vi "Profit Over Time v2.vi"() -> ()   [LabVIEW 2021]
uses:
  35c3a2be-d524-4b83-ae7a-0e43d7c29fc6.vi
  <vilib>/Array/Sort 2D Array - Pop Stack.vi
  <vilib>/Array/Sort 2D Array - Push Stack.vi
  35c3a2be-d524-4b83-ae7a-0e43d7c29fc6.vi/269d4b3b-47f5-49e3-8884-44851e4dd9d5.vi
  35c3a2be-d524-4b83-ae7a-0e43d7c29fc6.vi/6d99389c-673d-4efb-bf33-19b32bcf4cf8.vi
panel:
  in  "Export List?":bool
  in  "Go":bool
  in  "End Date":u16(ring) items=["Mon, Mar 22, 2021", "Mon, Mar 29, 2021", "Mon, Apr 5, 2021", "Mon, Apr 12, 2021", "Mon, Apr 19, 2021", "Mon, Apr 26, 2021", "Mon, May 3, 2021", "Tue, May 4, 2021", "Mon, May 10, 2021", "Mon, May 17, 2021", "Mon, May 24, 2021", "Mon, May 31, 2021", "Mon, Jun 7, 2021", "Mon, Jun 14, 2021", "Mon, Jun 21, 2021", "Mon, Jun 28, 2021", "Mon, Jul 5, 2021", "Mon, Jul 12, 2021", "Mon, Jul 19, 2021", "Mon, Jul 26, 2021", "Mon, Aug 2, 2021", "Mon, Aug 9, 2021", "Mon, Aug 16, 2021", "Mon, Aug 23, 2021", "Mon, Aug 30, 2021", "Mon, Sep 13, 2021", "Mon, Sep 20, 2021", "Mon, Sep 27, 2021", "Mon, Oct 4, 2021", "Mon, Oct 11, 2021", "Mon, Oct 18, 2021", "Mon, Nov 1, 2021", "Mon, Nov 8, 2021", "Mon, Nov 15, 2021", "Wed, Nov 24, 2021", "Mon, Nov 29, 2021", "Mon, Dec 6, 2021", "Mon, Dec 13, 2021", "Tue, Dec 14, 2021", "Wed, Dec 15, 2021", "Thu, Dec 16, 2021", "Fri, Dec 17, 2021", "Sat, Dec 18, 2021", "Mon, Dec 20, 2021", "Tue, Dec 28, 2021", "Wed, Dec 29, 2021", "Thu, Dec 30, 2021", "Fri, Dec 31, 2021", "Sat, Jan 1, 2022", "Sun, Jan 2, 2022", "Mon, Jan 3, 2022", "Tue, Jan 4, 2022", "Wed, Jan 5, 2022", "Thu, Jan 6, 2022", "Fri, Jan 7, 2022", "Sat, Jan 8, 2022", "Sun, Jan 9, 2022", "Mon, Jan 10, 2022", "Thu, Jan 13, 2022", "Sat, Jan 15, 2022", "Sun, Jan 16, 2022", "Mon, Jan 17, 2022", "Fri, Jan 21, 2022", "Mon, Jan 24, 2022", "Wed, Jan 26, 2022", "Thu, Jan 27, 2022", "Fri, Jan 28, 2022", "Sat, Jan 29, 2022", "Mon, Jan 31, 2022", "Wed, Feb 2, 2022", "Thu, Feb 3, 2022", "Mon, Feb 7, 2022", "Tue, Feb 8, 2022", "Wed, Feb 9, 2022", "Thu, Feb 10, 2022", "Fri, Feb 11, 2022", "Mon, Feb 14, 2022", "Tue, Feb 15, 2022", "Wed, Feb 16, 2022", "Thu, Feb 17, 2022", "Sun, Feb 20, 2022", "Mon, Feb 21, 2022", "Tue, Feb 22, 2022", "Wed, Feb 23, 2022", "Thu, Feb 24, 2022", "Fri, Feb 25, 2022", "Sat, Feb 26, 2022", "Sun, Feb 27, 2022", "Mon, Feb 28, 2022", "Fri, Mar 4, 2022", "Sat, Mar 5, 2022", "Sun, Mar 6, 2022", "Mon, Mar 7, 2022", "Tue, Mar 8, 2022", "Wed, Mar 9, 2022", "Fri, Mar 11, 2022", "Sat, Mar 12, 2022", "Sun, Mar 13, 2022", "Mon, Mar 14, 2022", "Wed, Mar 16, 2022", "Sat, Mar 19, 2022", "Sun, Mar 20, 2022", "Mon, Mar 21, 2022", "Tue, Mar 22, 2022", "Wed, Mar 23, 2022", "Thu, Mar 24, 2022", "Fri, Mar 25, 2022", "Sat, Mar 26, 2022", "Sun, Mar 27, 2022", "Mon, Mar 28, 2022", "Tue, Mar 29, 2022", "Wed, Mar 30, 2022", "Thu, Mar 31, 2022", "Sat, Apr 2, 2022", "Mon, Apr 4, 2022", "Sat, Apr 9, 2022", "Sun, Apr 10, 2022", "Mon, Apr 11, 2022", "Tue, Apr 12, 2022", "Wed, Apr 13, 2022", "Sat, Apr 16, 2022", "Sun, Apr 17, 2022", "Mon, Apr 18, 2022", "Thu, Apr 21, 2022", "Sat, Apr 23, 2022", "Sun, Apr 24, 2022", "Mon, Apr 25, 2022", "Tue, Apr 26, 2022", "Thu, Apr 28, 2022", "Fri, Apr 29, 2022", "Sat, Apr 30, 2022", "Mon, May 2, 2022", "Tue, May 3, 2022", "Wed, May 4, 2022", "Thu, May 5, 2022", "Fri, May 6, 2022", "Sat, May 7, 2022", "Sun, May 8, 2022", "Mon, May 9, 2022", "Wed, May 11, 2022", "Thu, May 12, 2022", "Fri, May 13, 2022", "Sat, May 14, 2022", "Sun, May 15, 2022", "Mon, May 16, 2022", "Tue, May 17, 2022", "Thu, May 19, 2022", "Fri, May 20, 2022", "Sat, May 21, 2022", "Sun, May 22, 2022", "Mon, May 23, 2022", "Tue, May 24, 2022", "Wed, May 25, 2022", "Thu, May 26, 2022", "Fri, May 27, 2022", "Sat, May 28, 2022", "Sun, May 29, 2022", "Mon, May 30, 2022", "Tue, May 31, 2022", "Wed, Jun 1, 2022", "Thu, Jun 2, 2022", "Fri, Jun 3, 2022", "Sat, Jun 4, 2022", "Sun, Jun 5, 2022", "Mon, Jun 6, 2022", "Tue, Jun 7, 2022", "Wed, Jun 8, 2022", "Thu, Jun 9, 2022", "Fri, Jun 10, 2022", "Sat, Jun 11, 2022", "Sun, Jun 12, 2022", "Mon, Jun 13, 2022", "Tue, Jun 14, 2022", "Wed, Jun 15, 2022", "Thu, Jun 16, 2022", "Fri, Jun 17, 2022", "Sat, Jun 18, 2022", "Sun, Jun 19, 2022", "Mon, Jun 20, 2022", "Tue, Jun 21, 2022", "Wed, Jun 22, 2022", "Thu, Jun 23, 2022", "Fri, Jun 24, 2022", "Sat, Jun 25, 2022", "Sun, Jun 26, 2022", "Mon, Jun 27, 2022", "Tue, Jun 28, 2022", "Fri, Jul 1, 2022", "Sat, Jul 2, 2022", "Sun, Jul 3, 2022", "Mon, Jul 4, 2022", "Tue, Jul 5, 2022", "Wed, Jul 6, 2022", "Thu, Jul 7, 2022", "Fri, Jul 8, 2022", "Sat, Jul 9, 2022", "Sun, Jul 10, 2022", "Mon, Jul 11, 2022", "Tue, Jul 12, 2022", "Wed, Jul 13, 2022", "Thu, Jul 14, 2022", "Fri, Jul 15, 2022", "Sat, Jul 16, 2022", "Fri, Jul 29, 2022", "Sat, Jul 30, 2022", "Mon, Aug 1, 2022", "Tue, Aug 2, 2022", "Wed, Aug 3, 2022", "Thu, Aug 4, 2022", "Fri, Aug 5, 2022", "Sat, Aug 6, 2022", "Sun, Aug 7, 2022", "Mon, Aug 8, 2022", "Tue, Aug 9, 2022", "Wed, Aug 10, 2022", "Thu, Aug 11, 2022", "Fri, Aug 12, 2022", "Sat, Aug 13, 2022", "Sun, Aug 14, 2022", "Mon, Aug 15, 2022", "Tue, Aug 16, 2022", "Wed, Aug 17, 2022", "Thu, Aug 18, 2022", "Fri, Aug 19, 2022", "Sat, Aug 20, 2022", "Sun, Aug 21, 2022", "Mon, Aug 22, 2022", "Tue, Aug 23, 2022", "Wed, Aug 24, 2022", "Thu, Aug 25, 2022", "Fri, Aug 26, 2022", "Sat, Aug 27, 2022", "Sun, Aug 28, 2022", "Mon, Aug 29, 2022", "Tue, Aug 30, 2022", "Wed, Aug 31, 2022", "Thu, Sep 1, 2022", "Fri, Sep 2, 2022", "Sat, Sep 3, 2022", "Sun, Sep 4, 2022", "Mon, Sep 5, 2022", "Tue, Sep 6, 2022", "Wed, Sep 7, 2022", "Sat, Sep 10, 2022", "Sun, Sep 11, 2022", "Mon, Sep 12, 2022", "Tue, Sep 13, 2022", "Wed, Sep 14, 2022", "Thu, Sep 15, 2022", "Fri, Sep 16, 2022", "Sat, Sep 17, 2022", "Sun, Sep 18, 2022", "Mon, Sep 19, 2022", "Tue, Sep 20, 2022", "Wed, Sep 21, 2022", "Thu, Sep 22, 2022", "Fri, Sep 23, 2022", "Sat, Sep 24, 2022", "Sun, Sep 25, 2022", "Mon, Sep 26, 2022", "Tue, Sep 27, 2022", "Wed, Sep 28, 2022", "Thu, Sep 29, 2022", "Fri, Sep 30, 2022", "Sat, Oct 1, 2022", "Mon, Oct 3, 2022", "Wed, Oct 5, 2022", "Thu, Oct 6, 2022", "Fri, Oct 7, 2022", "Sat, Oct 8, 2022", "Mon, Oct 10, 2022", "Wed, Oct 12, 2022", "Thu, Oct 13, 2022", "Fri, Oct 14, 2022", "Sat, Oct 15, 2022", "Mon, Oct 17, 2022", "Tue, Oct 18, 2022", "Wed, Oct 19, 2022", "Thu, Oct 20, 2022", "Fri, Oct 21, 2022", "Sat, Oct 22, 2022", "Sun, Oct 23, 2022", "Mon, Oct 24, 2022", "Tue, Oct 25, 2022", "Wed, Oct 26, 2022", "Thu, Oct 27, 2022", "Fri, Oct 28, 2022", "Sat, Oct 29, 2022", "Mon, Oct 31, 2022", "Tue, Nov 1, 2022", "Wed, Nov 2, 2022", "Thu, Nov 3, 2022", "Fri, Nov 4, 2022", "Sat, Nov 5, 2022", "Sun, Nov 6, 2022", "Mon, Nov 7, 2022", "Wed, Nov 9, 2022", "Thu, Nov 10, 2022", "Fri, Nov 11, 2022", "Sat, Nov 12, 2022", "Sun, Nov 13, 2022", "Mon, Nov 14, 2022", "Tue, Nov 15, 2022", "Thu, Nov 17, 2022", "Fri, Nov 18, 2022", "Sat, Nov 19, 2022", "Mon, Nov 21, 2022", "Tue, Nov 22, 2022", "Wed, Nov 23, 2022", "Thu, Nov 24, 2022", "Fri, Nov 25, 2022", "Sat, Nov 26, 2022", "Sun, Nov 27, 2022", "Mon, Nov 28, 2022", "Tue, Nov 29, 2022", "Wed, Nov 30, 2022", "Thu, Dec 1, 2022", "Fri, Dec 2, 2022", "Tue, Dec 13, 2022", "Wed, Dec 14, 2022", "Thu, Dec 15, 2022", "Fri, Dec 16, 2022", "Sat, Dec 17, 2022", "Sun, Dec 18, 2022", "Mon, Dec 19, 2022", "Tue, Dec 20, 2022", "Wed, Dec 21, 2022", "Thu, Dec 22, 2022", "Fri, Dec 23, 2022", "Sat, Dec 24, 2022", "Sun, Dec 25, 2022", "Mon, Dec 26, 2022", "Tue, Dec 27, 2022", "Wed, Dec 28, 2022", "Thu, Dec 29, 2022", "Fri, Dec 30, 2022", "Sat, Dec 31, 2022", "Sun, Jan 1, 2023", "Mon, Jan 2, 2023"]
  in  "Start Date":u16(ring) items=["Mon, Mar 22, 2021", "Mon, Mar 29, 2021", "Mon, Apr 5, 2021", "Mon, Apr 12, 2021", "Mon, Apr 19, 2021", "Mon, Apr 26, 2021", "Mon, May 3, 2021", "Tue, May 4, 2021", "Mon, May 10, 2021", "Mon, May 17, 2021", "Mon, May 24, 2021", "Mon, May 31, 2021", "Mon, Jun 7, 2021", "Mon, Jun 14, 2021", "Mon, Jun 21, 2021", "Mon, Jun 28, 2021", "Mon, Jul 5, 2021", "Mon, Jul 12, 2021", "Mon, Jul 19, 2021", "Mon, Jul 26, 2021", "Mon, Aug 2, 2021", "Mon, Aug 9, 2021", "Mon, Aug 16, 2021", "Mon, Aug 23, 2021", "Mon, Aug 30, 2021", "Mon, Sep 13, 2021", "Mon, Sep 20, 2021", "Mon, Sep 27, 2021", "Mon, Oct 4, 2021", "Mon, Oct 11, 2021", "Mon, Oct 18, 2021", "Mon, Nov 1, 2021", "Mon, Nov 8, 2021", "Mon, Nov 15, 2021", "Wed, Nov 24, 2021", "Mon, Nov 29, 2021", "Mon, Dec 6, 2021", "Mon, Dec 13, 2021", "Tue, Dec 14, 2021", "Wed, Dec 15, 2021", "Thu, Dec 16, 2021", "Fri, Dec 17, 2021", "Sat, Dec 18, 2021", "Mon, Dec 20, 2021", "Tue, Dec 28, 2021", "Wed, Dec 29, 2021", "Thu, Dec 30, 2021", "Fri, Dec 31, 2021", "Sat, Jan 1, 2022", "Sun, Jan 2, 2022", "Mon, Jan 3, 2022", "Tue, Jan 4, 2022", "Wed, Jan 5, 2022", "Thu, Jan 6, 2022", "Fri, Jan 7, 2022", "Sat, Jan 8, 2022", "Sun, Jan 9, 2022", "Mon, Jan 10, 2022", "Thu, Jan 13, 2022", "Sat, Jan 15, 2022", "Sun, Jan 16, 2022", "Mon, Jan 17, 2022", "Fri, Jan 21, 2022", "Mon, Jan 24, 2022", "Wed, Jan 26, 2022", "Thu, Jan 27, 2022", "Fri, Jan 28, 2022", "Sat, Jan 29, 2022", "Mon, Jan 31, 2022", "Wed, Feb 2, 2022", "Thu, Feb 3, 2022", "Mon, Feb 7, 2022", "Tue, Feb 8, 2022", "Wed, Feb 9, 2022", "Thu, Feb 10, 2022", "Fri, Feb 11, 2022", "Mon, Feb 14, 2022", "Tue, Feb 15, 2022", "Wed, Feb 16, 2022", "Thu, Feb 17, 2022", "Sun, Feb 20, 2022", "Mon, Feb 21, 2022", "Tue, Feb 22, 2022", "Wed, Feb 23, 2022", "Thu, Feb 24, 2022", "Fri, Feb 25, 2022", "Sat, Feb 26, 2022", "Sun, Feb 27, 2022", "Mon, Feb 28, 2022", "Fri, Mar 4, 2022", "Sat, Mar 5, 2022", "Sun, Mar 6, 2022", "Mon, Mar 7, 2022", "Tue, Mar 8, 2022", "Wed, Mar 9, 2022", "Fri, Mar 11, 2022", "Sat, Mar 12, 2022", "Sun, Mar 13, 2022", "Mon, Mar 14, 2022", "Wed, Mar 16, 2022", "Sat, Mar 19, 2022", "Sun, Mar 20, 2022", "Mon, Mar 21, 2022", "Tue, Mar 22, 2022", "Wed, Mar 23, 2022", "Thu, Mar 24, 2022", "Fri, Mar 25, 2022", "Sat, Mar 26, 2022", "Sun, Mar 27, 2022", "Mon, Mar 28, 2022", "Tue, Mar 29, 2022", "Wed, Mar 30, 2022", "Thu, Mar 31, 2022", "Sat, Apr 2, 2022", "Mon, Apr 4, 2022", "Sat, Apr 9, 2022", "Sun, Apr 10, 2022", "Mon, Apr 11, 2022", "Tue, Apr 12, 2022", "Wed, Apr 13, 2022", "Sat, Apr 16, 2022", "Sun, Apr 17, 2022", "Mon, Apr 18, 2022", "Thu, Apr 21, 2022", "Sat, Apr 23, 2022", "Sun, Apr 24, 2022", "Mon, Apr 25, 2022", "Tue, Apr 26, 2022", "Thu, Apr 28, 2022", "Fri, Apr 29, 2022", "Sat, Apr 30, 2022", "Mon, May 2, 2022", "Tue, May 3, 2022", "Wed, May 4, 2022", "Thu, May 5, 2022", "Fri, May 6, 2022", "Sat, May 7, 2022", "Sun, May 8, 2022", "Mon, May 9, 2022", "Wed, May 11, 2022", "Thu, May 12, 2022", "Fri, May 13, 2022", "Sat, May 14, 2022", "Sun, May 15, 2022", "Mon, May 16, 2022", "Tue, May 17, 2022", "Thu, May 19, 2022", "Fri, May 20, 2022", "Sat, May 21, 2022", "Sun, May 22, 2022", "Mon, May 23, 2022", "Tue, May 24, 2022", "Wed, May 25, 2022", "Thu, May 26, 2022", "Fri, May 27, 2022", "Sat, May 28, 2022", "Sun, May 29, 2022", "Mon, May 30, 2022", "Tue, May 31, 2022", "Wed, Jun 1, 2022", "Thu, Jun 2, 2022", "Fri, Jun 3, 2022", "Sat, Jun 4, 2022", "Sun, Jun 5, 2022", "Mon, Jun 6, 2022", "Tue, Jun 7, 2022", "Wed, Jun 8, 2022", "Thu, Jun 9, 2022", "Fri, Jun 10, 2022", "Sat, Jun 11, 2022", "Sun, Jun 12, 2022", "Mon, Jun 13, 2022", "Tue, Jun 14, 2022", "Wed, Jun 15, 2022", "Thu, Jun 16, 2022", "Fri, Jun 17, 2022", "Sat, Jun 18, 2022", "Sun, Jun 19, 2022", "Mon, Jun 20, 2022", "Tue, Jun 21, 2022", "Wed, Jun 22, 2022", "Thu, Jun 23, 2022", "Fri, Jun 24, 2022", "Sat, Jun 25, 2022", "Sun, Jun 26, 2022", "Mon, Jun 27, 2022", "Tue, Jun 28, 2022", "Fri, Jul 1, 2022", "Sat, Jul 2, 2022", "Sun, Jul 3, 2022", "Mon, Jul 4, 2022", "Tue, Jul 5, 2022", "Wed, Jul 6, 2022", "Thu, Jul 7, 2022", "Fri, Jul 8, 2022", "Sat, Jul 9, 2022", "Sun, Jul 10, 2022", "Mon, Jul 11, 2022", "Tue, Jul 12, 2022", "Wed, Jul 13, 2022", "Thu, Jul 14, 2022", "Fri, Jul 15, 2022", "Sat, Jul 16, 2022", "Fri, Jul 29, 2022", "Sat, Jul 30, 2022", "Mon, Aug 1, 2022", "Tue, Aug 2, 2022", "Wed, Aug 3, 2022", "Thu, Aug 4, 2022", "Fri, Aug 5, 2022", "Sat, Aug 6, 2022", "Sun, Aug 7, 2022", "Mon, Aug 8, 2022", "Tue, Aug 9, 2022", "Wed, Aug 10, 2022", "Thu, Aug 11, 2022", "Fri, Aug 12, 2022", "Sat, Aug 13, 2022", "Sun, Aug 14, 2022", "Mon, Aug 15, 2022", "Tue, Aug 16, 2022", "Wed, Aug 17, 2022", "Thu, Aug 18, 2022", "Fri, Aug 19, 2022", "Sat, Aug 20, 2022", "Sun, Aug 21, 2022", "Mon, Aug 22, 2022", "Tue, Aug 23, 2022", "Wed, Aug 24, 2022", "Thu, Aug 25, 2022", "Fri, Aug 26, 2022", "Sat, Aug 27, 2022", "Sun, Aug 28, 2022", "Mon, Aug 29, 2022", "Tue, Aug 30, 2022", "Wed, Aug 31, 2022", "Thu, Sep 1, 2022", "Fri, Sep 2, 2022", "Sat, Sep 3, 2022", "Sun, Sep 4, 2022", "Mon, Sep 5, 2022", "Tue, Sep 6, 2022", "Wed, Sep 7, 2022", "Sat, Sep 10, 2022", "Sun, Sep 11, 2022", "Mon, Sep 12, 2022", "Tue, Sep 13, 2022", "Wed, Sep 14, 2022", "Thu, Sep 15, 2022", "Fri, Sep 16, 2022", "Sat, Sep 17, 2022", "Sun, Sep 18, 2022", "Mon, Sep 19, 2022", "Tue, Sep 20, 2022", "Wed, Sep 21, 2022", "Thu, Sep 22, 2022", "Fri, Sep 23, 2022", "Sat, Sep 24, 2022", "Sun, Sep 25, 2022", "Mon, Sep 26, 2022", "Tue, Sep 27, 2022", "Wed, Sep 28, 2022", "Thu, Sep 29, 2022", "Fri, Sep 30, 2022", "Sat, Oct 1, 2022", "Mon, Oct 3, 2022", "Wed, Oct 5, 2022", "Thu, Oct 6, 2022", "Fri, Oct 7, 2022", "Sat, Oct 8, 2022", "Mon, Oct 10, 2022", "Wed, Oct 12, 2022", "Thu, Oct 13, 2022", "Fri, Oct 14, 2022", "Sat, Oct 15, 2022", "Mon, Oct 17, 2022", "Tue, Oct 18, 2022", "Wed, Oct 19, 2022", "Thu, Oct 20, 2022", "Fri, Oct 21, 2022", "Sat, Oct 22, 2022", "Sun, Oct 23, 2022", "Mon, Oct 24, 2022", "Tue, Oct 25, 2022", "Wed, Oct 26, 2022", "Thu, Oct 27, 2022", "Fri, Oct 28, 2022", "Sat, Oct 29, 2022", "Mon, Oct 31, 2022", "Tue, Nov 1, 2022", "Wed, Nov 2, 2022", "Thu, Nov 3, 2022", "Fri, Nov 4, 2022", "Sat, Nov 5, 2022", "Sun, Nov 6, 2022", "Mon, Nov 7, 2022", "Wed, Nov 9, 2022", "Thu, Nov 10, 2022", "Fri, Nov 11, 2022", "Sat, Nov 12, 2022", "Sun, Nov 13, 2022", "Mon, Nov 14, 2022", "Tue, Nov 15, 2022", "Thu, Nov 17, 2022", "Fri, Nov 18, 2022", "Sat, Nov 19, 2022", "Mon, Nov 21, 2022", "Tue, Nov 22, 2022", "Wed, Nov 23, 2022", "Thu, Nov 24, 2022", "Fri, Nov 25, 2022", "Sat, Nov 26, 2022", "Sun, Nov 27, 2022", "Mon, Nov 28, 2022", "Tue, Nov 29, 2022", "Wed, Nov 30, 2022", "Thu, Dec 1, 2022", "Fri, Dec 2, 2022", "Tue, Dec 13, 2022", "Wed, Dec 14, 2022", "Thu, Dec 15, 2022", "Fri, Dec 16, 2022", "Sat, Dec 17, 2022", "Sun, Dec 18, 2022", "Mon, Dec 19, 2022", "Tue, Dec 20, 2022", "Wed, Dec 21, 2022", "Thu, Dec 22, 2022", "Fri, Dec 23, 2022", "Sat, Dec 24, 2022", "Sun, Dec 25, 2022", "Mon, Dec 26, 2022", "Tue, Dec 27, 2022", "Wed, Dec 28, 2022", "Thu, Dec 29, 2022", "Fri, Dec 30, 2022", "Sat, Dec 31, 2022", "Sun, Jan 1, 2023", "Mon, Jan 2, 2023"]
  out "Complete List":cluster{"Player Name":string, "Profit":dbl}[](array[cluster])
  out "Top 5":cluster{"Player Name":string, "Profit":dbl}[](array[cluster])
  out "residual":dbl
  in  "file path (use dialog)":path=path "C:/Users/manma/Google Drive/WPC Stat Scrape/Data/WPC Stats.bin"
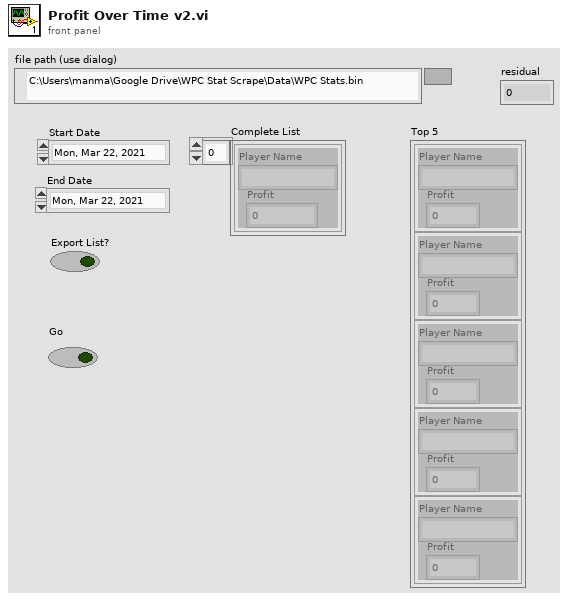
[diagram p1: front panel]
types:
  T1 = typedef "WPC Player and Financial Stats.ctl" = cluster{"Player Name":string, "Date Updated":timestamp, "Tournament Stats":cluster{"Hands Won":i32, "Hands Played":i32, "Hands Dealt":i32, "All-Ins":i32, "Entered":i32, "Winnings":dbl, "Profit":dbl}, "Cash Stats":cluster{"Hands Won":i32, "Hands Played":i32, "Hands Dealt":i32, "All-Ins":i32, "Profit":dbl}}
  T2 = enum16{"open", "replace", "create", "open or create", "replace or create", "replace or create with confirmation"}
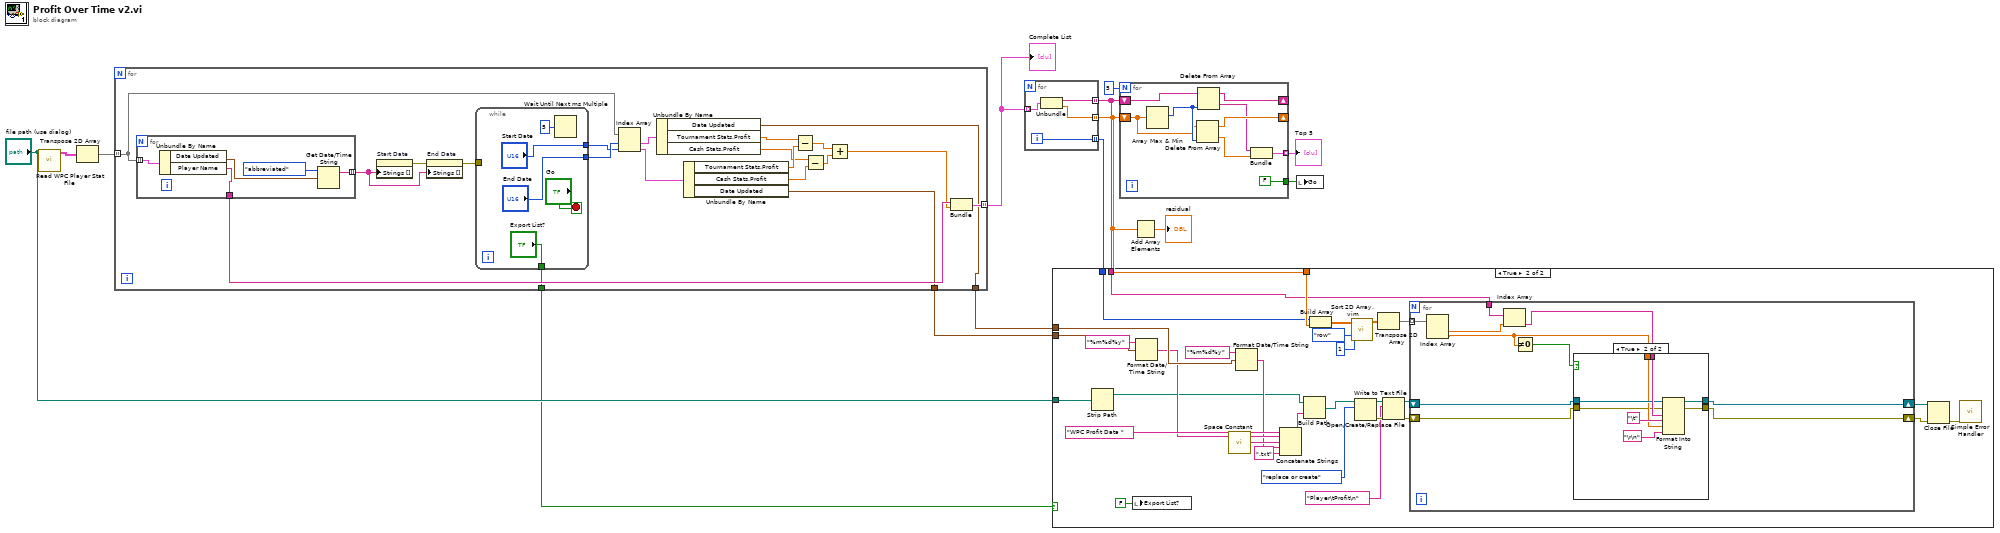
[diagram p0: block diagram]
diagram:
  n1 = call "Read WPC Player Stat File.vi"("file path (use dialog)"="file path (use dialog)") -> ("Full WPC Stats"=w13:T1[][])  [unwired: 8 in, 2 out]
  n2 = Transpose 2D Array(2D array=w13) -> (transposed array=w14:T1[][])
  n3 = for {
    tunnel: w14 -> [w29] mode=indexing
    tunnel: [w34] -> w10 mode=indexing
    tunnel: [w17] -> w3
    tunnel: [w16] -> w2
    tunnel: [w15] -> w1
    n4 = for {
      tunnel: w29 -> [w40] mode=indexing
      tunnel: [w44] -> w33
      tunnel: [w41] -> w31 mode=indexing
      n5 = Unbundle By Name(w40) -> ("Date Updated"=w43:timestamp, "Player Name"=w44:string)
      n6 = Get Date/Time String(date format (0)=enum16{"short", "long", "abbreviated"}."abbreviated", seconds (now)=w43) -> (date string=w41:string)  [unwired: 1 in, 1 out]
    }
    n7 = property on="Start Date" class="Ring (strict)"("Strings []"=w31) -> (error out=w32:errorcluster)  [unwired: 2 in, 1 out]
    n8 = property on="End Date" class="Ring (strict)"(error in=w32, "Strings []"=w31) -> (error out=w30:errorcluster)  [unwired: 1 in, 1 out]
    n9 = while {
      tunnel: w30 -> [_]
      tunnel: ["Start Date"] -> w27
      tunnel: ["End Date"] -> w28
      tunnel: ["Export List?"] -> w15
      stop <- "Go" stop-if-true
      n10 = Wait Until Next ms Multiple(millisecond multiple=u32 5) -> ()  [unwired: 1 out]
    }
    n11 = Index Array(array=w29, index #1=w28, index #2=w27) -> (element #1=w26:T1, element #2=w25:T1)
    n12 = Unbundle By Name(w26) -> ("Date Updated"=w16:timestamp, "Tournament Stats.Profit"=w24:dbl, "Cash Stats.Profit"=w22:dbl)
    n13 = Unbundle By Name(w25) -> ("Tournament Stats.Profit"=w23:dbl, "Cash Stats.Profit"=w21:dbl, "Date Updated"=w17:timestamp)
    n14 = Subtract(x=w24, y=w23) -> (x-y=w19:dbl)
    n15 = Subtract(x=w22, y=w21) -> (x-y=w20:dbl)
    n16 = Add(x=w19, y=w20) -> (x+y=w18:dbl)
    n17 = Bundle("Player Name"=w33, w18) -> (w34:cluster{"Player Name":string, dbl})  [unwired: 1 in]
  }
  "Complete List" <- w10
  n18 = for {
    tunnel: w10 -> [w48] mode=indexing
    tunnel: [w47] -> w5 mode=indexing
    tunnel: [w46] -> w7 mode=indexing
    tunnel: [w45] -> w6 mode=indexing
    i -> [w45]
    n19 = Unbundle(w48) -> ("Player Name"=w47:string, w46:dbl)
  }
  n20 = case shown="True" w1 {
    tunnel: w7 -> [_ w79]
    tunnel: w6 -> [_ w78]
    tunnel: w5 -> [_ w73]
    tunnel: "file path (use dialog)" -> [_ w71]
    tunnel: w3 -> [_ w70]
    tunnel: w2 -> [_ w67]
    frame False {
    }
    frame True {
      n21 = Strip Path(path=w71) -> (stripped path=w59:path)  [unwired: 1 out]
      n22 = local write "Export List?"(FALSE ("Export List?")) -> ()
      n23 = Format Date/Time String(time format string (%c)="%m%d%y", seconds (now)=w70) -> (date/time string=w65:string)  [unwired: 1 in]
      n24 = call <vilib>:"Space Constant.vi"() -> ("String"=w64:string)
      n25 = Format Date/Time String(time format string (%c)="%m%d%y", seconds (now)=w67) -> (date/time string=w63:string)  [unwired: 1 in]
      n26 = Concatenate Strings("WPC Profit Data ", w65, w64, w63, ".txt" ("string")) -> (w60:string)
      n27 = Build Path(base path=w59, name or relative path=w60) -> (appended path=w61:path)
      n28 = Build Array(w78, w79) -> (w77:dbl[][])
      n29 = call "Sort 2D Array.vim"("index"=1, "dimension to index (column)"=enum16{"column", "row"}."row", "2D array"=w77) -> ("sorted 2D array"=w74:dbl[][])  [unwired: 7 in, 1 out]
      n30 = Open/Create/Replace File(file path (use dialog)=w61, operation (0:open)=T2."replace or create") -> (refnum out=w57:refnum<file>, error out=w56:errorcluster)  [unwired: 4 in, 1 out]
      n31 = Transpose 2D Array(2D array=w74) -> (transposed array=w72:dbl[][])
      n32 = Write to Text File(file (use dialog)=w57, text="Player\tProfit\n", error in=w56) -> (refnum out=w53:refnum<file>, error out=w54:errorcluster)  [unwired: 1 in, 1 out]
      n33 = for {
        tunnel: w72 -> [w89] mode=indexing
        tunnel: w73 -> [w88]
        shift-right: [w81] -> w51
        shift-left: w54 -> [w83]
        shift-right: [w82] -> w52
        shift-left: w53 -> [w85]
        n34 = Index Array(array=w89) -> (element #1=w87:dbl, element #2=w84:dbl)  [unwired: 2 in]
        n35 = Index Array(array=w88, index=w87) -> (element=w86:string)
        n36 = Not Equal To 0?(x=w84) -> (x != 0?=w80:bool)
        n37 = case shown="True" w80 {
          tunnel: w86 -> [_ w99]
          tunnel: w85 -> [w91 w98]
          tunnel: w84 -> [_ w96]
          tunnel: w83 -> [w90 w95]
          tunnel: [w90 w93] -> w81
          tunnel: [w91 w92] -> w82
          frame False {
          }
          frame True {
            n38 = Format Into String(initial string=w98, error in=w95, w99, "\t", w96, "\r\n") -> (resulting string=w92:refnum<file>, error out=w93:errorcluster)  [unwired: 1 in]
          }
        }
      }
      n39 = Close File(refnum=w52, error in=w51) -> (error out=w50:errorcluster)  [unwired: 1 out]
      n40 = call <vilib>:"Simple Error Handler.vi"("error in (no error)"=w50) -> ()  [unwired: 4 in, 5 out]
    }
  }
  n41 = for {
    N: 5 -> [_]
    shift-right: [w106] -> _
    shift-left: w7 -> [w101]
    shift-right: [w107] -> _
    shift-left: w5 -> [w102]
    tunnel: [w103] -> w9 mode=indexing
    tunnel: [FALSE] -> w8
    n42 = Array Max & Min(array=w101) -> (max index (indices)=w108:i32)  [unwired: 3 out]
    n43 = Delete From Array(array=w101, index=w108) -> (deleted portion=w104:dbl, array with subset deleted=w106:dbl[])  [unwired: 1 in]
    n44 = Delete From Array(array=w102, index=w108) -> (deleted portion=w105:string, array with subset deleted=w107:string[])  [unwired: 1 in]
    n45 = Bundle("Player Name"=w105, w104) -> (w103:cluster{"Player Name":string, dbl})  [unwired: 1 in]
  }
  "Top 5" <- w9
  n46 = Add Array Elements(numeric array=w7) -> (sum=→"residual":dbl)
  n47 = local write "Go"(w8) -> ()
